vi "Speech Controlled Robot.vi"() -> ()   [LabVIEW 2022 SP3]
uses:
  <vilib>/LabVIEW Interface for Arduino/Type Defs/Pin Mode.ctl
  <vilib>/LabVIEW Interface for Arduino/LabVIEW Interface for Arduino.lvlib
panel:
  out "Executable Commands":string
  in  "VISA Resource Port":refnum<visa-resource-name>
  in  "Exit":bool caption="Stop Execution"
  out "Recognised Command":string
  # "SPEECH CONTROLLED ROBOT"
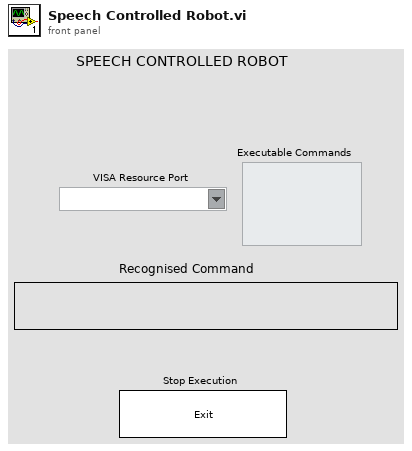
[diagram p1: front panel]
types:
  T1 = typedef "LabVIEW Interface for Arduino.lvlib/Arduino Resource.ctl" = cluster{"VISA resource":refnum<visa-resource-name>, "Board Type":T2, "Connection Type":enum8{"USB / Serial"}, "Bytes Per Packet (15)":u8}
  T2 = typedef "LabVIEW Interface for Arduino.lvlib/Board Type.ctl" = enum16{"Uno", "Dimuelanove w/Atmega 328", "Mega 2560"}
  T3 = typedef "LabVIEW Interface for Arduino.lvlib/Pin Mode.ctl" = enum8{"Input", "Output"}
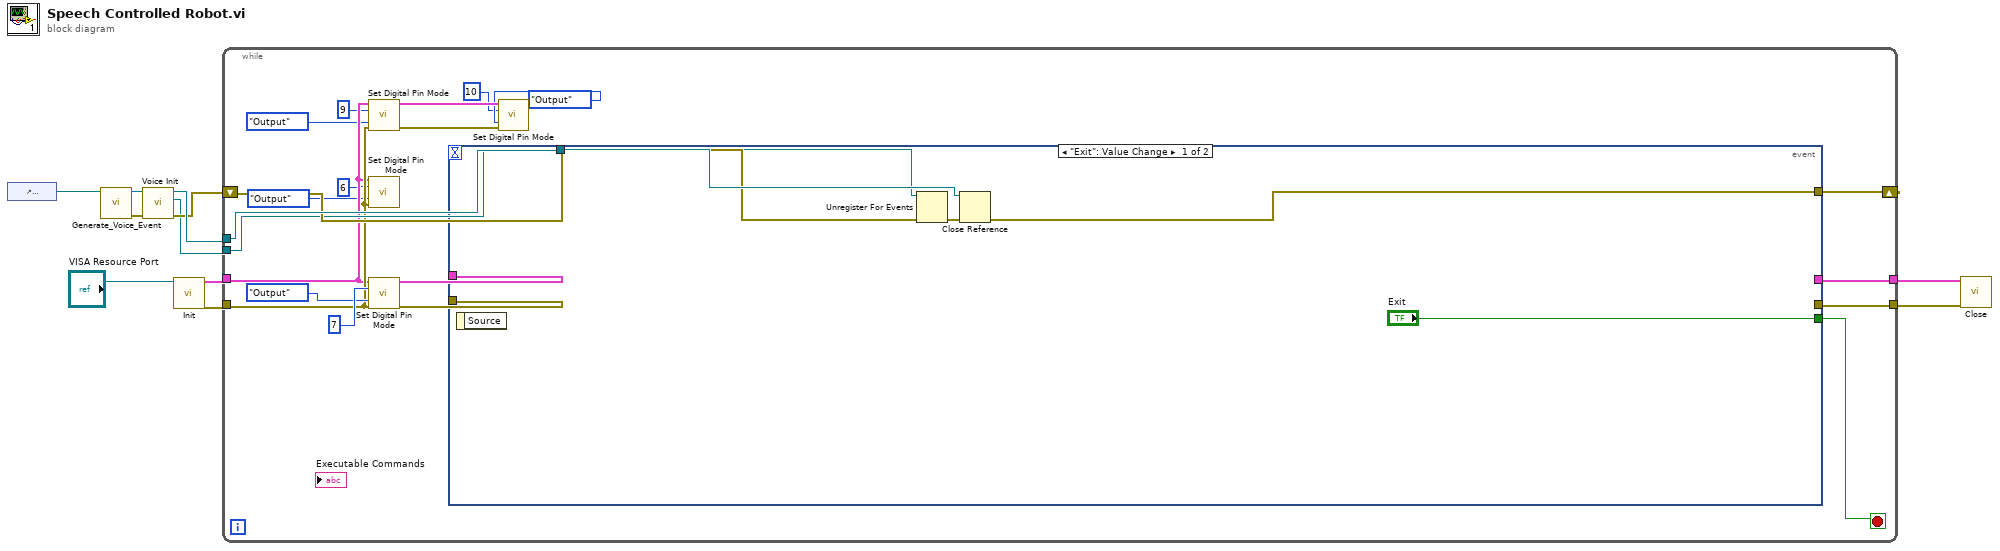
[diagram p0: block diagram]
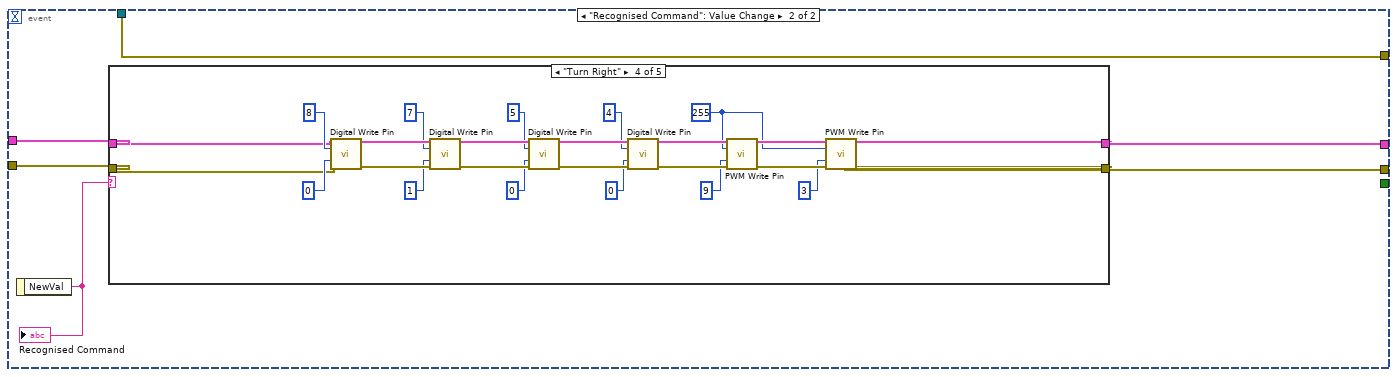
[diagram p2: hidden frame]
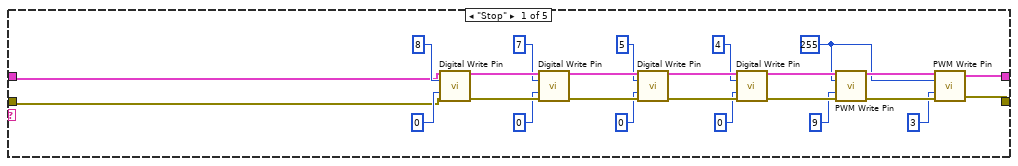
[diagram p3: hidden frame]
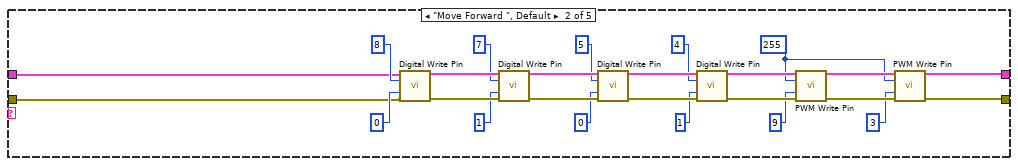
[diagram p4: hidden frame]
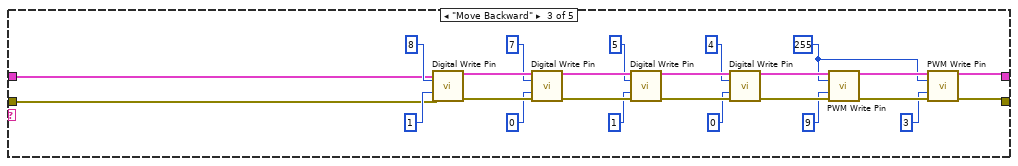
[diagram p5: hidden frame]
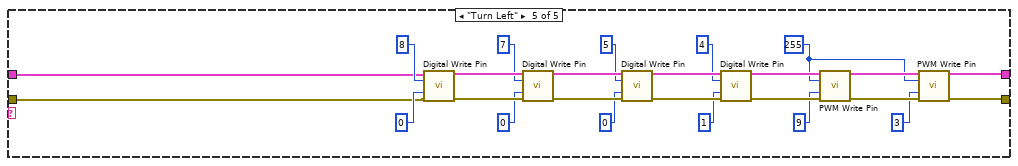
[diagram p6: hidden frame]
diagram:
  n1 = control-ref of="Recognised Command"() -> (w10:refnum<vi>)
  n2 = call "Generate_Voice_Event.vi"("String in"=w10) -> ("Error Out"=w9:errorcluster, "String out"=w11:refnum<vi>)  [unwired: 9 in]
  n3 = call "Voice Init.vi"("Error In"=w9, "Text"=w11) -> ("Error Out"=w7:errorcluster, "Event Callback"=w6:refnum<k27>, "Reference"=w8:refnum<k24>)  [unwired: 7 in]
  n4 = call <vilib>:"Init.vi"("VISA resource"="VISA Resource Port") -> ("Arduino Resource"=w3:T1, "error out"=w2:errorcluster)  [unwired: 17 in]
  n5 = while {
    tunnel: w8 -> [w32]
    shift-right: [w30] -> _
    shift-left: w7 -> [w31]
    tunnel: w6 -> [w29]
    tunnel: w3 -> [w19]
    tunnel: w2 -> [w20]
    tunnel: [w26] -> w4
    tunnel: [w25] -> w5
    stop <- w12 stop-if-true
    n6 = call <vilib>:"Set Digital Pin Mode.vi"("Arduino Resource"=w19, "Digital I/O Pin"=u8 9, "Pin Mode (Input)"=Pin_Mode."Output", "error in"=w20) -> ("Arduino Resource"=w22:T1, "error out"=w21:errorcluster)  [unwired: 10 in]
    n7 = call <vilib>:"Set Digital Pin Mode.vi"("Arduino Resource"=w19, "Digital I/O Pin"=u8 6, "Pin Mode (Input)"=Pin_Mode."Output", "error in"=w20) -> ()  [unwired: 10 in, 2 out]
    n8 = call <vilib>:"Set Digital Pin Mode.vi"("Arduino Resource"=w19, "Digital I/O Pin"=u8 7, "Pin Mode (Input)"=Pin_Mode."Output", "error in"=w20) -> ("Arduino Resource"=w28:T1, "error out"=w27:errorcluster)  [unwired: 10 in]
    n9 = event shown="[0] \"Exit\": Value Change" {
      selector: _ -> [_ _]
      dyn-events: _ -> [_ _]
      timeout: _ -> [_ _]
      tunnel: w32 -> [w38 _]
      tunnel: w31 -> [w36 w44]
      tunnel: [w35 w44] -> w30
      tunnel: w29 -> [w34 _]
      tunnel: w28 -> [_ w42]
      tunnel: w27 -> [_ w41]
      tunnel: [_ w39] -> w26
      tunnel: [_ w40] -> w25
      tunnel: ["Exit" _] -> w12
      event "Exit": Value Change {
        n10 = event-data() -> ()  [unwired: 1 in, 1 out]
        n11 = Unregister For Events(event registration refnum=w34, error in=w36) -> (error out=w37:errorcluster)
        n12 = Close Reference(reference=w38, error in (no error)=w37) -> (error out=w35:errorcluster)
      }
      event "Recognised Command": Value Change {
        n13 = event-data() -> ("NewVal"=w43:string)  [unwired: 1 in]
        "Recognised Command" <- w43
        n14 = case shown="\"Turn Right\"" w43 {
          tunnel: w42 -> [w48 w73 w98 w121 w148]
          tunnel: w41 -> [w47 w72 w97 w120 w147]
          tunnel: [w45 w70 w95 w122 w145] -> w40
          tunnel: [w46 w71 w96 w123 w146] -> w39
          frame "Stop" {
            w55 = u8 255 ("Duty Cycle (0 - 255)")
            n15 = call <vilib>:"Digital Write Pin.vi"("Arduino Resource"=w48, "Digital I/O Pin (0)"=u8 8, "Value (0)"=u8 0, "error in"=w47) -> ("Arduino Resource"=w61:T1, "error out"=w60:errorcluster)  [unwired: 10 in]
            n16 = call <vilib>:"Digital Write Pin.vi"("Arduino Resource"=w61, "Digital I/O Pin (0)"=u8 7, "Value (0)"=u8 0, "error in"=w60) -> ("Arduino Resource"=w64:T1, "error out"=w65:errorcluster)  [unwired: 10 in]
            n17 = call <vilib>:"Digital Write Pin.vi"("Arduino Resource"=w64, "Digital I/O Pin (0)"=u8 5, "Value (0)"=u8 0, "error in"=w65) -> ("Arduino Resource"=w66:T1, "error out"=w67:errorcluster)  [unwired: 10 in]
            n18 = call <vilib>:"Digital Write Pin.vi"("Arduino Resource"=w66, "Digital I/O Pin (0)"=u8 4, "Value (0)"=u8 0, "error in"=w67) -> ("Arduino Resource"=w68:T1, "error out"=w69:errorcluster)  [unwired: 10 in]
            n19 = call <vilib>:"PWM Write Pin.vi"("Arduino Resource"=w68, "Duty Cycle (0 - 255)"=w55, "PWM Pin (3)"=u8 9, "error in"=w69) -> ("Arduino Resource"=w62:T1, "error out"=w63:errorcluster)  [unwired: 10 in]
            n20 = call <vilib>:"PWM Write Pin.vi"("Arduino Resource"=w62, "Duty Cycle (0 - 255)"=w55, "PWM Pin (3)"=u8 3, "error in"=w63) -> ("Arduino Resource"=w46:T1, "error out"=w45:errorcluster)  [unwired: 10 in]
          }
          frame "Move Forward ", Default {
            w76 = u8 255 ("Duty Cycle (0 - 255)")
            n21 = call <vilib>:"Digital Write Pin.vi"("Arduino Resource"=w73, "Digital I/O Pin (0)"=u8 8, "Value (0)"=u8 0, "error in"=w72) -> ("Arduino Resource"=w93:T1, "error out"=w94:errorcluster)  [unwired: 10 in]
            n22 = call <vilib>:"Digital Write Pin.vi"("Arduino Resource"=w93, "Digital I/O Pin (0)"=u8 7, "Value (0)"=u8 1, "error in"=w94) -> ("Arduino Resource"=w90:T1, "error out"=w89:errorcluster)  [unwired: 10 in]
            n23 = call <vilib>:"Digital Write Pin.vi"("Arduino Resource"=w90, "Digital I/O Pin (0)"=u8 5, "Value (0)"=u8 0, "error in"=w89) -> ("Arduino Resource"=w88:T1, "error out"=w87:errorcluster)  [unwired: 10 in]
            n24 = call <vilib>:"Digital Write Pin.vi"("Arduino Resource"=w88, "Digital I/O Pin (0)"=u8 4, "Value (0)"=u8 1, "error in"=w87) -> ("Arduino Resource"=w86:T1, "error out"=w85:errorcluster)  [unwired: 10 in]
            n25 = call <vilib>:"PWM Write Pin.vi"("Arduino Resource"=w86, "Duty Cycle (0 - 255)"=w76, "PWM Pin (3)"=u8 9, "error in"=w85) -> ("Arduino Resource"=w92:T1, "error out"=w91:errorcluster)  [unwired: 10 in]
            n26 = call <vilib>:"PWM Write Pin.vi"("Arduino Resource"=w92, "Duty Cycle (0 - 255)"=w76, "PWM Pin (3)"=u8 3, "error in"=w91) -> ("Arduino Resource"=w71:T1, "error out"=w70:errorcluster)  [unwired: 10 in]
          }
          frame "Move Backward" {
            w101 = u8 255 ("Duty Cycle (0 - 255)")
            n27 = call <vilib>:"Digital Write Pin.vi"("Arduino Resource"=w98, "Digital I/O Pin (0)"=u8 8, "Value (0)"=u8 1, "error in"=w97) -> ("Arduino Resource"=w118:T1, "error out"=w119:errorcluster)  [unwired: 10 in]
            n28 = call <vilib>:"Digital Write Pin.vi"("Arduino Resource"=w118, "Digital I/O Pin (0)"=u8 7, "Value (0)"=u8 0, "error in"=w119) -> ("Arduino Resource"=w115:T1, "error out"=w114:errorcluster)  [unwired: 10 in]
            n29 = call <vilib>:"Digital Write Pin.vi"("Arduino Resource"=w115, "Digital I/O Pin (0)"=u8 5, "Value (0)"=u8 1, "error in"=w114) -> ("Arduino Resource"=w113:T1, "error out"=w112:errorcluster)  [unwired: 10 in]
            n30 = call <vilib>:"Digital Write Pin.vi"("Arduino Resource"=w113, "Digital I/O Pin (0)"=u8 4, "Value (0)"=u8 0, "error in"=w112) -> ("Arduino Resource"=w111:T1, "error out"=w110:errorcluster)  [unwired: 10 in]
            n31 = call <vilib>:"PWM Write Pin.vi"("Arduino Resource"=w111, "Duty Cycle (0 - 255)"=w101, "PWM Pin (3)"=u8 9, "error in"=w110) -> ("Arduino Resource"=w117:T1, "error out"=w116:errorcluster)  [unwired: 10 in]
            n32 = call <vilib>:"PWM Write Pin.vi"("Arduino Resource"=w117, "Duty Cycle (0 - 255)"=w101, "PWM Pin (3)"=u8 3, "error in"=w116) -> ("Arduino Resource"=w96:T1, "error out"=w95:errorcluster)  [unwired: 10 in]
          }
          frame "Turn Right" {
            w130 = u8 255 ("Duty Cycle (0 - 255)")
            n33 = call <vilib>:"Digital Write Pin.vi"("Arduino Resource"=w121, "Digital I/O Pin (0)"=u8 8, "Value (0)"=u8 0, "error in"=w120) -> ("Arduino Resource"=w136:T1, "error out"=w135:errorcluster)  [unwired: 10 in]
            n34 = call <vilib>:"Digital Write Pin.vi"("Arduino Resource"=w136, "Digital I/O Pin (0)"=u8 7, "Value (0)"=u8 1, "error in"=w135) -> ("Arduino Resource"=w139:T1, "error out"=w140:errorcluster)  [unwired: 10 in]
            n35 = call <vilib>:"Digital Write Pin.vi"("Arduino Resource"=w139, "Digital I/O Pin (0)"=u8 5, "Value (0)"=u8 0, "error in"=w140) -> ("Arduino Resource"=w141:T1, "error out"=w142:errorcluster)  [unwired: 10 in]
            n36 = call <vilib>:"Digital Write Pin.vi"("Arduino Resource"=w141, "Digital I/O Pin (0)"=u8 4, "Value (0)"=u8 0, "error in"=w142) -> ("Arduino Resource"=w143:T1, "error out"=w144:errorcluster)  [unwired: 10 in]
            n37 = call <vilib>:"PWM Write Pin.vi"("Arduino Resource"=w143, "Duty Cycle (0 - 255)"=w130, "PWM Pin (3)"=u8 9, "error in"=w144) -> ("Arduino Resource"=w137:T1, "error out"=w138:errorcluster)  [unwired: 10 in]
            n38 = call <vilib>:"PWM Write Pin.vi"("Arduino Resource"=w137, "Duty Cycle (0 - 255)"=w130, "PWM Pin (3)"=u8 3, "error in"=w138) -> ("Arduino Resource"=w123:T1, "error out"=w122:errorcluster)  [unwired: 10 in]
          }
          frame "Turn Left" {
            w151 = u8 255 ("Duty Cycle (0 - 255)")
            n39 = call <vilib>:"Digital Write Pin.vi"("Arduino Resource"=w148, "Digital I/O Pin (0)"=u8 8, "Value (0)"=u8 0, "error in"=w147) -> ("Arduino Resource"=w168:T1, "error out"=w169:errorcluster)  [unwired: 10 in]
            n40 = call <vilib>:"Digital Write Pin.vi"("Arduino Resource"=w168, "Digital I/O Pin (0)"=u8 7, "Value (0)"=u8 0, "error in"=w169) -> ("Arduino Resource"=w165:T1, "error out"=w164:errorcluster)  [unwired: 10 in]
            n41 = call <vilib>:"Digital Write Pin.vi"("Arduino Resource"=w165, "Digital I/O Pin (0)"=u8 5, "Value (0)"=u8 0, "error in"=w164) -> ("Arduino Resource"=w163:T1, "error out"=w162:errorcluster)  [unwired: 10 in]
            n42 = call <vilib>:"Digital Write Pin.vi"("Arduino Resource"=w163, "Digital I/O Pin (0)"=u8 4, "Value (0)"=u8 1, "error in"=w162) -> ("Arduino Resource"=w161:T1, "error out"=w160:errorcluster)  [unwired: 10 in]
            n43 = call <vilib>:"PWM Write Pin.vi"("Arduino Resource"=w161, "Duty Cycle (0 - 255)"=w151, "PWM Pin (3)"=u8 9, "error in"=w160) -> ("Arduino Resource"=w167:T1, "error out"=w166:errorcluster)  [unwired: 10 in]
            n44 = call <vilib>:"PWM Write Pin.vi"("Arduino Resource"=w167, "Duty Cycle (0 - 255)"=w151, "PWM Pin (3)"=u8 3, "error in"=w166) -> ("Arduino Resource"=w146:T1, "error out"=w145:errorcluster)  [unwired: 10 in]
          }
        }
      }
    }
    n45 = call <vilib>:"Set Digital Pin Mode.vi"("Arduino Resource"=w22, "Digital I/O Pin"=u8 10, "Pin Mode (Input)"=Pin_Mode."Output", "error in"=w21) -> ()  [unwired: 10 in, 2 out]
  }
  n46 = call <vilib>:"Close.vi"("Arduino Resource"=w4, "error in"=w5) -> ()  [unwired: 13 in, 1 out]
